vi "createNewArrayObject.vi"(8 "error in (no error)":errorcluster, 10 "arrayRef":refnum<vi>, 11 "Primitive in":refnum<class "Primitive.lvclass">) -> (0 "error out":errorcluster, 3 "Primitive out":refnum<class "Primitive.lvclass">)   [LabVIEW 2016, in "Primitive.lvclass"]
uses:
  Primitive.lvclass
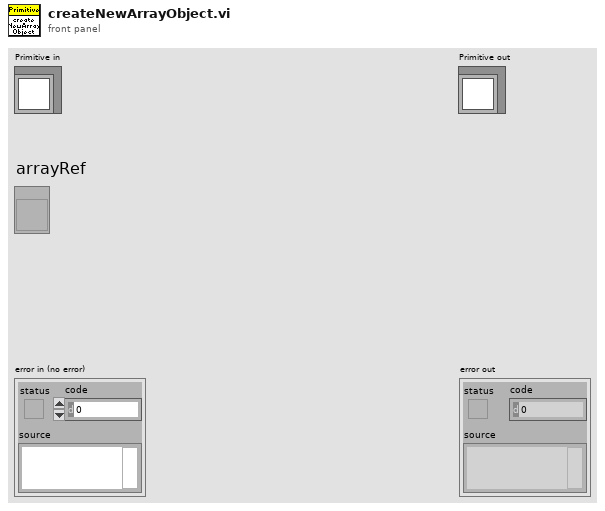
[diagram p1: front panel]
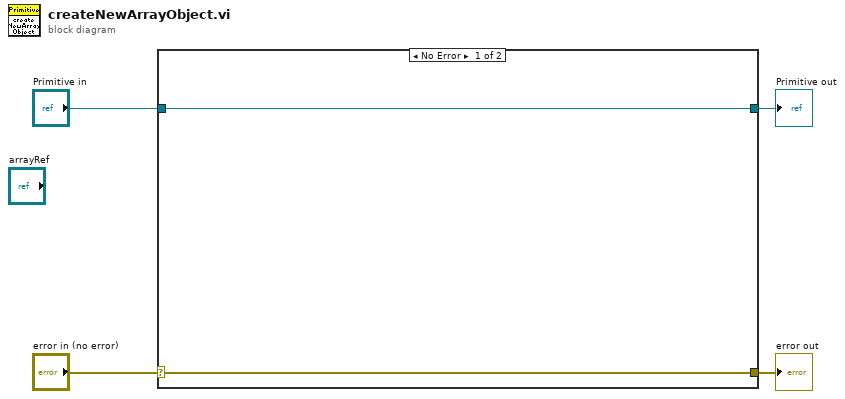
[diagram p0: block diagram]
diagram:
  n1 = case shown="No Error" "error in (no error)" {
    selector: "error in (no error)" -> [w5 w8]
    tunnel: [w5 w8] -> w3
    tunnel: [w6 w7] -> w1
    tunnel: "Primitive in" -> [w6 w7]
    frame No Error {
    }
    frame Error {
    }
  }
  "error out" <- w3
  "Primitive out" <- w1
